vi "Translate Drive.vi"(7 "Translation PID Gains":T1={"proportional gain (Kc)"=1.0, "integral time (Ti, min)"=0.01, "derivative time (Td, min)"=0.0} {"derivative time (Td, min)" format="%.3f"; "integral time (Ti, min)" format="%.3f"; "proportional gain (Kc)" format="%.3f"}, 8 "Translation Tolerance":dbl, 9 "Z Min Output":dbl, 10 "Z Max Output":dbl, 11 "Target Translation":dbl) -> (0 "Finished?":bool, 1 "Z Out":dbl)   [LabVIEW 2016]
uses:
  Common Code/PID Gains.ctl
  Common Code/Utilities/Change Detect Double.vi
  <vilib>/addons/control/pid/pid.llb/PID (DBL).vi
  <vilib>/addons/control/pid/NI_PID_pid.lvlib
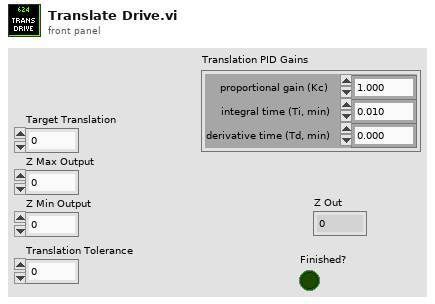
[diagram p1: front panel]
types:
  T1 = typedef "PID Gains.ctl" = cluster{"proportional gain (Kc)":dbl, "integral time (Ti, min)":dbl, "derivative time (Td, min)":dbl}
  T2 = typedef "Drivetrain Encoder Values.ctl" = cluster{"Left Encoder":T3, "Center Encoder":T3, "Right Encoder":T3}
  T3 = typedef "Encoder Values.ctl" = cluster{"Distance":dbl, "Speed":dbl, "Tick":dbl}
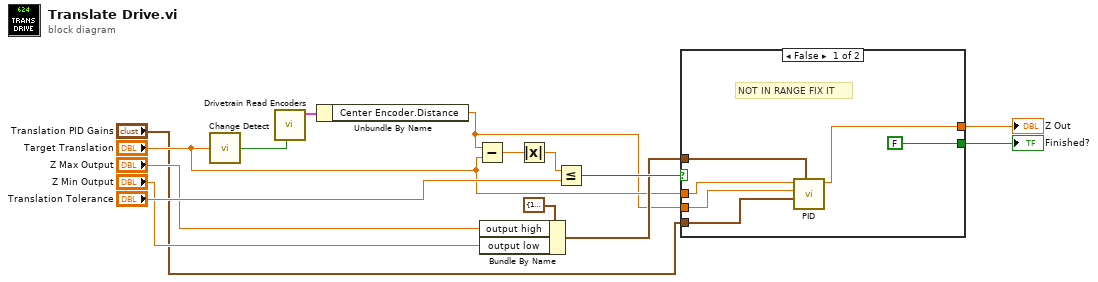
[diagram p0: block diagram]
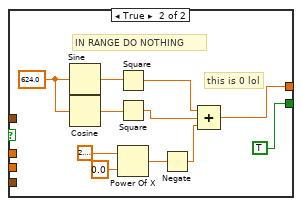
[diagram p2: hidden frame]
diagram:
  n1 = call-poly "Change Detect.vi"("In"="Target Translation") -> ("Changed?"=w15:bool)
  n2 = call "Drivetrain Read Encoders.vi"("Reset Encoders"=w15) -> ("Drivetrain Encoder Values"=w14:T2)  [unwired: 10 in]
  n3 = Unbundle By Name(w14) -> ("Center Encoder.Distance"=w4:dbl)
  n4 = Subtract(x=w4, y="Target Translation") -> (x-y=w13:dbl)
  n5 = Bundle By Name(cluster=cluster{"output high":dbl, "output low":dbl} {"output high"=100.0, "output low"=-100.0} ("output range"), "output high"="Z Max Output", "output low"="Z Min Output") -> (w6:cluster{"output high":dbl, "output low":dbl})
  n6 = Absolute Value(x=w13) -> (abs(x)=w12:dbl)
  n7 = Less Or Equal?(x=w12, y="Translation Tolerance") -> (x <= y?=w10:bool)
  n8 = case shown="False" w10 {
    tunnel: w6 -> [w21 _]
    tunnel: "Target Translation" -> [w20 _]
    tunnel: w4 -> [w19 _]
    tunnel: "Translation PID Gains" -> [w18 _]
    tunnel: [w17 w23] -> w2
    tunnel: [FALSE TRUE] -> w1
    frame False {
      # "NOT IN RANGE FIX IT"
      n9 = call-poly <vilib>:"PID.vi"("output range"=w21, "PID gains"=w18, "process variable"=w19, "setpoint"=w20) -> ("output"=w17:dbl)  [unwired: 6 in, 1 out]
    }
    frame True {
      w32 = 624.0 ("x")
      # "this is 0 lol"
      # "IN RANGE DO NOTHING"
      n10 = Sine(x=w32) -> (sin(x)=w31:dbl)
      n11 = Cosine(x=w32) -> (cos(x)=w30:dbl)
      n12 = Square(x=w31) -> (x^2=w29:dbl)
      n13 = Square(x=w30) -> (x^2=w28:dbl)
      n14 = Power Of X(1:0.0 ("x"), 2:2.718281828459045) -> (0:w25:dbl)
      n15 = Negate(x=w25) -> (-x=w24:dbl)
      n16 = Compound Arithmetic op=unknown(w29, w28, w24) -> (w23:dbl)
    }
  }
  "Z Out" <- w2
  "Finished?" <- w1
